vi "log_error.vi"(6 "timestamp":timestamp, 7 "context":string, 8 "error in (no error)":errorcluster, 9 "level":T1=200 items=["OFF"=0, "FATAL"=100, "ERROR"=200, "WARN"=300, "INFO"=400, "DEBUG"=500, "TRACE"=600, "ALL"=65535], 11 "Log Service in":refnum<class "Log Service.lvclass">) -> (0 "error out":errorcluster, 3 "Log Service out":refnum<class "Log Service.lvclass">)   [LabVIEW 2019, in "Utility API.lvlib" / "Log Service.lvclass"]
uses:
  Log Service.lvclass
  public/level.ctl
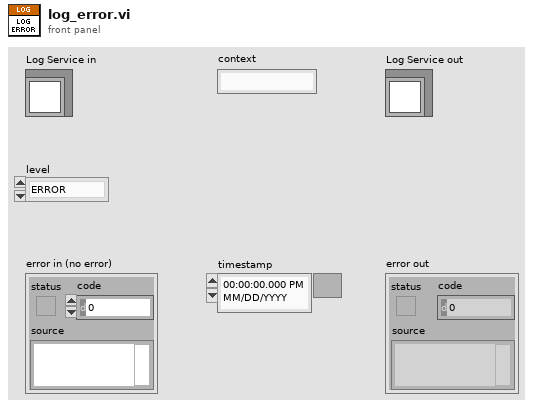
[diagram p1: front panel]
types:
  T1 = typedef "Utility API.lvlib/Log Service.lvclass/level.ctl" = u16
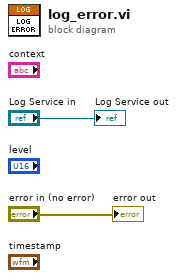
[diagram p0: block diagram]
diagram:
  "error out" <- "error in (no error)"
  "Log Service out" <- "Log Service in"
